vi "Delete Line.vi"(8 "error in":errorcluster, 10 "Active Line Name":string, 11 "Custom Temperature Controller configuration in":refnum<class "Custom Temperature Controller configuration.lvclass">) -> (0 "error out":errorcluster, 2 "Deleted Line":T1, 3 "Custom Temperature Controller configuration out":refnum<class "Custom Temperature Controller configuration.lvclass">)   [LabVIEW 2021, in "Custom Temperature Controller configuration.lvclass"]
uses:
  Custom Temperature Controller configuration.lvclass
  <vilib>/NI/Tag Bus Module Framework/channel/TBM channel.lvclass
  Custom Temperature Controller configuration.lvclass/Custom Temperature Controller configuration.ctl
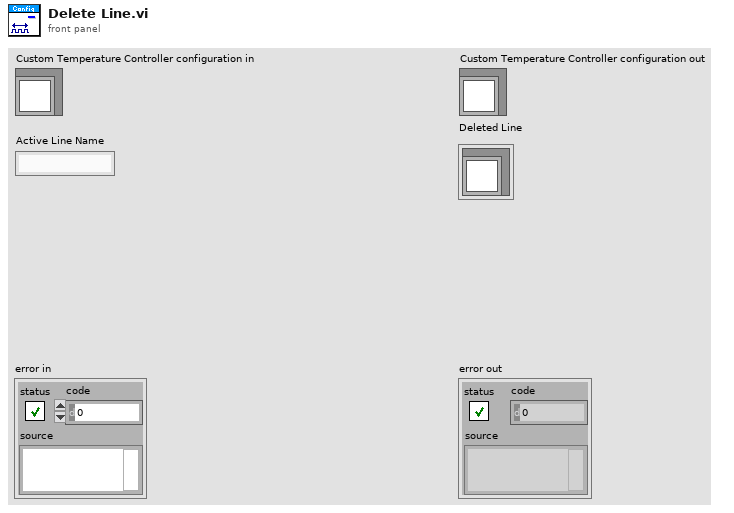
[diagram p1: front panel]
types:
  T1 = cluster{"channel":refnum<class "TBM channel.lvclass">}
  T2 = cluster{"channel":refnum<class "TBM channel.lvclass">}[]
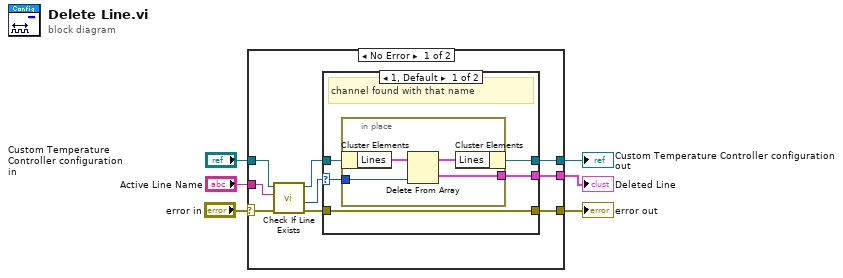
[diagram p0: block diagram]
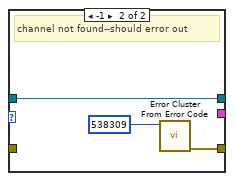
[diagram p2: hidden frame]
diagram:
  n1 = case shown="No Error" "error in" {
    selector: "error in" -> [w8 w29]
    tunnel: [w14 w29] -> w5
    tunnel: [w15 w28] -> w3
    tunnel: "Custom Temperature Controller configuration in" -> [w12 w28]
    tunnel: "Active Line Name" -> [w7 _]
    tunnel: [w13 _] -> w1
    frame No Error {
      n2 = call-dynamic "Check If Line Exists.vi"("error in (no error)"=w8, "name to locate"=w7, "Custom Temperature Controller configuration in"=w12) -> ("error out"=w9:errorcluster, "index"=w10:i32, "Custom Temperature Controller configuration out"=w11:refnum<class "Custom Temperature Controller configuration.lvclass">)  [unwired: 4 in, 2 out]
      n3 = case shown="1, Default" w10 {
        selector: w10 -> [w16 _]
        tunnel: [w18 w27] -> w14
        tunnel: w11 -> [w20 w25]
        tunnel: [w19 w25] -> w15
        tunnel: w9 -> [w18 _]
        tunnel: [w17 _] -> w13
        frame 1, Default {
          # "channel found with that name"
          n4 = in-place {
            in-place-border: w16 -> [w24]
            in-place-border: [w21] -> w17
            n5 = in-place-cluster #1(w20) -> ("Lines"=w23:T2)
            n6 = Delete From Array(array=w23, index=w24) -> (deleted portion=w21:T1, array with subset deleted=w22:T2)  [unwired: 1 in]
            n7 = in-place-cluster #1("Lines"=w22) -> (w19:refnum<class "Custom Temperature Controller configuration.lvclass">)
          }
        }
        frame -1 {
          # "channel not found--should error out"
          n8 = call <vilib>:"Error Cluster From Error Code.vi"("error code (0)"=538309) -> ("error out"=w27:errorcluster)  [unwired: 8 in]
        }
      }
    }
    frame Error {
    }
  }
  "error out" <- w5
  "Custom Temperature Controller configuration out" <- w3
  "Deleted Line" <- w1
